vi "Ch_data_pattern_8_save (SubVI).vi"(7 "error in":errorcluster, 14 "T Cluster":T1, 15 "Activate!":bool, 16 "R Cluster":T2, 17 "file":refnum<file>) -> (27 "error out":errorcluster)   [LabVIEW 2013]
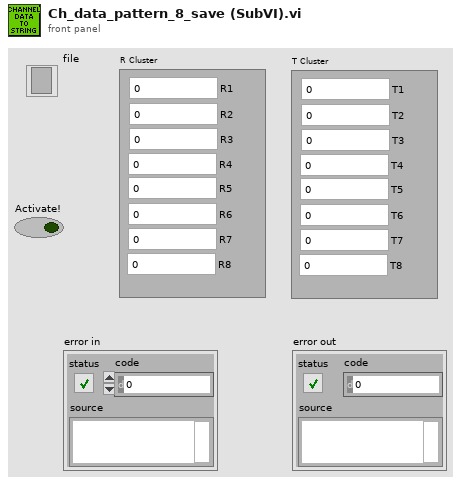
[diagram p1: front panel]
types:
  T1 = cluster{"T1":dbl, "T2":dbl, "T3":dbl, "T4":dbl, "T5":dbl, "T6":dbl, "T7":dbl, "T8":dbl}
  T2 = cluster{"R1":dbl, "R2":dbl, "R3":dbl, "R4":dbl, "R5":dbl, "R6":dbl, "R7":dbl, "R8":dbl}
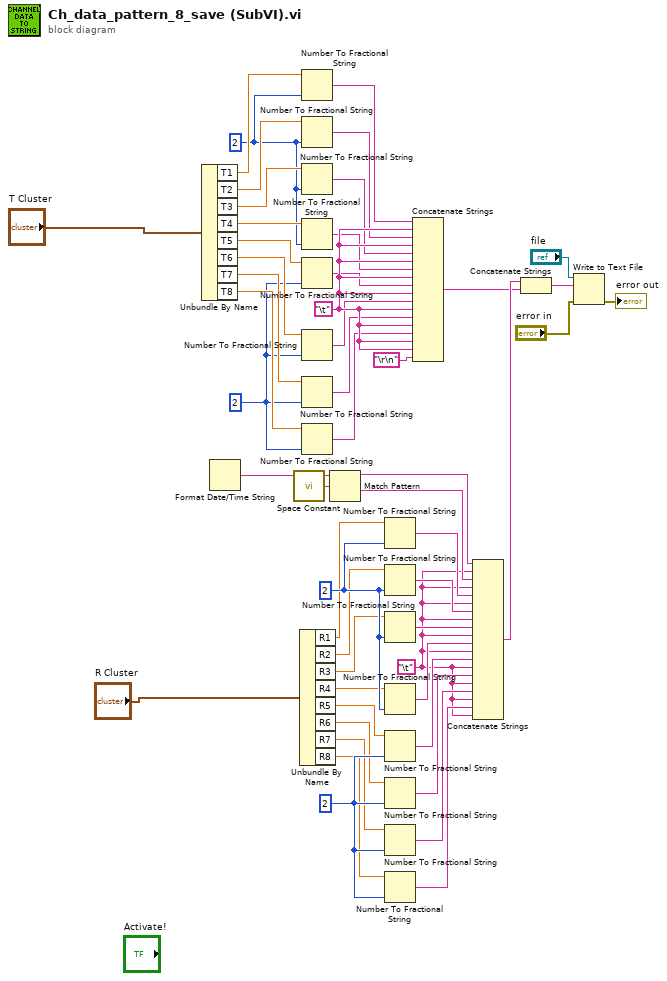
[diagram p0: block diagram]
diagram:
  w11 = i16 2 ("precision (6)")
  w7 = i16 2 ("precision (6)")
  w24 = "\t"
  w40 = i16 2 ("precision (6)")
  w50 = i16 2 ("precision (6)")
  w27 = "\t"
  n1 = Unbundle By Name("T Cluster") -> ("T1"=w16:dbl, "T2"=w17:dbl, "T3"=w18:dbl, "T4"=w19:dbl, "T5"=w20:dbl, "T6"=w21:dbl, "T7"=w22:dbl, "T8"=w23:dbl)
  n2 = Format Date/Time String() -> (date/time string=w42:string)  [unwired: 3 out]
  n3 = call <vilib>:"Space Constant.vi"() -> ("String"=w43:string)
  n4 = Unbundle By Name("R Cluster") -> ("R1"=w35:dbl, "R2"=w34:dbl, "R3"=w33:dbl, "R4"=w32:dbl, "R5"=w31:dbl, "R6"=w30:dbl, "R7"=w29:dbl, "R8"=w28:dbl)
  n5 = Number To Fractional String(number=w16, precision (6)=w7) -> (F-format string=w10:string)  [unwired: 2 out]
  n6 = Number To Fractional String(number=w17, precision (6)=w7) -> (F-format string=w3:string)  [unwired: 2 out]
  n7 = Number To Fractional String(number=w18, precision (6)=w7) -> (F-format string=w9:string)  [unwired: 2 out]
  n8 = Number To Fractional String(number=w19, precision (6)=w7) -> (F-format string=w8:string)  [unwired: 2 out]
  n9 = Number To Fractional String(number=w20, precision (6)=w11) -> (F-format string=w12:string)  [unwired: 2 out]
  n10 = Number To Fractional String(number=w21, precision (6)=w11) -> (F-format string=w13:string)  [unwired: 2 out]
  n11 = Number To Fractional String(number=w22, precision (6)=w11) -> (F-format string=w14:string)  [unwired: 2 out]
  n12 = Number To Fractional String(number=w23, precision (6)=w11) -> (F-format string=w15:string)  [unwired: 2 out]
  n13 = Match Pattern(string=w42, regular expression=w43) -> (before substring=w44:string, after substring=w45:string)  [unwired: 3 out]
  n14 = Number To Fractional String(number=w35, precision (6)=w50) -> (F-format string=w46:string)  [unwired: 2 out]
  n15 = Number To Fractional String(number=w34, precision (6)=w50) -> (F-format string=w47:string)  [unwired: 2 out]
  n16 = Number To Fractional String(number=w33, precision (6)=w50) -> (F-format string=w48:string)  [unwired: 2 out]
  n17 = Number To Fractional String(number=w32, precision (6)=w50) -> (F-format string=w49:string)  [unwired: 2 out]
  n18 = Number To Fractional String(number=w31, precision (6)=w40) -> (F-format string=w39:string)  [unwired: 2 out]
  n19 = Number To Fractional String(number=w30, precision (6)=w40) -> (F-format string=w38:string)  [unwired: 2 out]
  n20 = Number To Fractional String(number=w29, precision (6)=w40) -> (F-format string=w37:string)  [unwired: 2 out]
  n21 = Number To Fractional String(number=w28, precision (6)=w40) -> (F-format string=w36:string)  [unwired: 2 out]
  n22 = Concatenate Strings(w10, w24, w3, w24, w9, w24, w8, w24, w12, w24, w13, w24, w14, w24, w15, w24, w24, "\r\n") -> (w5:string)
  n23 = Concatenate Strings(w44, w27, w45, w27, w46, w27, w47, w27, w48, w27, w49, w27, w39, w27, w38, w27, w37, w27, w36, w27) -> (w26:string)
  n24 = Concatenate Strings(w26, w5) -> (w25:string)
  n25 = Write to Text File(file (use dialog)="file", text=w25, error in="error in") -> (error out=→"error out":errorcluster)  [unwired: 3 out]
